vi "Translate Raw Data.vi"(8 "Error In":errorcluster, 10 "Raw Weather Data":T4, 11 "Open Weather Session In":refnum<class "Open Weather Session.lvclass">) -> (0 "Error Out":errorcluster, 2 "Weather Data":T1, 3 "Open Weather Session Out":refnum<class "Open Weather Session.lvclass">)   [LabVIEW 2019, in "Open Weather Session.lvclass"]
uses:
  Open Weather Session.lvclass
  Controls/Raw Weather Data.ctl
  Controls/Weather Sample Raw Data.ctl
  Controls/Weather Description Raw Data.ctl
  Public/Controls/Weather Data.ctl
  Public/Controls/Weather Sample Data.ctl
  Public/Controls/Weather Description Data.ctl
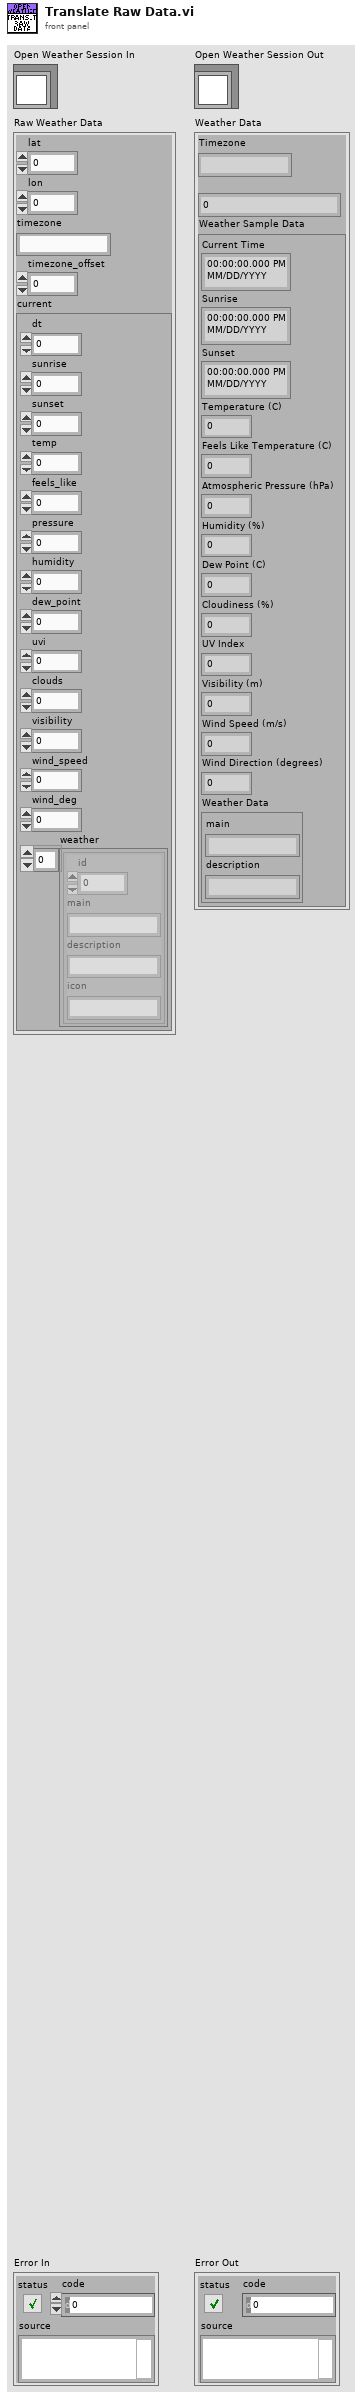
[diagram p1: front panel]
types:
  T1 = typedef "Open Weather Session.lvclass/Weather Data.ctl" = cluster{"Timezone":string, "Timezone Offset":dbl, "Weather Sample Data":T2}
  T2 = typedef "Open Weather Session.lvclass/Weather Sample Data.ctl" = cluster{"Current Time":timestamp, "Sunrise":timestamp, "Sunset":timestamp, "Temperature (C)":dbl, "Feels Like Temperature (C)":dbl, "Atmospheric Pressure (hPa)":dbl, "Humidity (%)":dbl, "Dew Point (C)":dbl, "Cloudiness (%)":dbl, "UV Index":dbl, "Visibility (m)":dbl, "Wind Speed (m/s)":dbl, "Wind Direction (degrees)":dbl, "Weather Data":T3}
  T3 = typedef "Open Weather Session.lvclass/Weather Description Data.ctl" = cluster{"main":string, "description":string}
  T4 = typedef "Open Weather Session.lvclass/Raw Weather Data.ctl" = cluster{"lat":dbl, "lon":dbl, "timezone":string, "timezone_offset":dbl, "current":T5}
  T5 = typedef "Open Weather Session.lvclass/Weather Sample Raw Data.ctl" = cluster{"dt":dbl, "sunrise":dbl, "sunset":dbl, "temp":dbl, "feels_like":dbl, "pressure":i32, "humidity":i32, "dew_point":dbl, "uvi":dbl, "clouds":i32, "visibility":i32, "wind_speed":dbl, "wind_deg":i32, "weather":T6[]}
  T6 = typedef "Open Weather Session.lvclass/Weather Description Raw Data.ctl" = cluster{"id":u32, "main":string, "description":string, "icon":string}
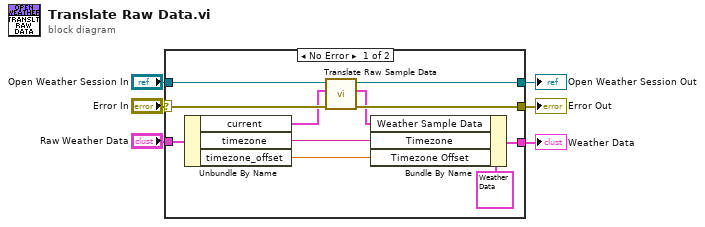
[diagram p0: block diagram]
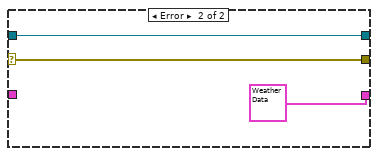
[diagram p2: hidden frame]
diagram:
  n1 = case shown="No Error" "Error In" {
    selector: "Error In" -> [w14 w19]
    tunnel: [w15 w20] -> w6
    tunnel: [w13 w19] -> w5
    tunnel: "Open Weather Session In" -> [w16 w20]
    tunnel: "Raw Weather Data" -> [w17 _]
    tunnel: [w9 T1 {"Timezone"="", "Timezone Offset"=0.0, "Weather Sample Data"={"Current Time"=timestamp(0 s since 1904-01-01), "Sunrise"=timestamp(0 s since 1904-01-01), "Sunset"=timestamp(0 s since 1904-01-01), "Temperature (C)"=0.0, "Feels Like Temperature (C)"=0.0, "Atmospheric Pressure (hPa)"=0.0, "Humidity (%)"=0.0, "Dew Point (C)"=0.0, "Cloudiness (%)"=0.0, "UV Index"=0.0, "Visibility (m)"=0.0, "Wind Speed (m/s)"=0.0, "Wind Direction (degrees)"=0.0, "Weather Data"={"main"="", "description"=""}}} ("Weather Data")] -> w1
    frame No Error {
      n2 = Unbundle By Name(w17) -> ("current"=w12:T5, "timezone"=w10:string, "timezone_offset"=w7:dbl)
      n3 = call "Translate Raw Sample Data.vi"("Error In"=w14, "Sample Raw Data"=w12, "Open Weather Session In"=w16) -> ("Error Out"=w13:errorcluster, "Weather Sample Data"=w8:T2, "Open Weather Session Out"=w15:refnum<class "Open Weather Session.lvclass">)  [unwired: 6 in]
      n4 = Bundle By Name(cluster=T1 {"Timezone"="", "Timezone Offset"=0.0, "Weather Sample Data"={"Current Time"=timestamp(0 s since 1904-01-01), "Sunrise"=timestamp(0 s since 1904-01-01), "Sunset"=timestamp(0 s since 1904-01-01), "Temperature (C)"=0.0, "Feels Like Temperature (C)"=0.0, "Atmospheric Pressure (hPa)"=0.0, "Humidity (%)"=0.0, "Dew Point (C)"=0.0, "Cloudiness (%)"=0.0, "UV Index"=0.0, "Visibility (m)"=0.0, "Wind Speed (m/s)"=0.0, "Wind Direction (degrees)"=0.0, "Weather Data"={"main"="", "description"=""}}} ("Weather Data"), "Weather Sample Data"=w8, "Timezone"=w10, "Timezone Offset"=w7) -> (w9:T1)
    }
    frame Error {
    }
  }
  "Open Weather Session Out" <- w6
  "Error Out" <- w5
  "Weather Data" <- w1
